vi "Stop Acquisition.vi"(0 "fpga interface in":refnum<k20>, 9 "timeout (s)":dbl=20.0 format="%#_13g", 11 "error in (no error)":errorcluster) -> (4 "fpga interface out":refnum<k20>, 15 "error out":errorcluster)   [LabVIEW 2023, in "GettingStarted_Acq_148X_Host.lvlib"]
uses:
  GettingStarted_Acq_148X_Host.lvlib
  <instrlib>/FlexRIO/CSI-2/v2/FPGA/Types/Global Acquisition Engine State.ctl
  Types/148x_Acq_FPGA_Reference.ctl
  <vilib>/Utility/error.llb/Error Cluster From Error Code.vi
  <vilib>/rvi/errors/niLvFpgaAdjustHostInterfaceError.vi
  <vilib>/rvi/interface/nirviReadWriteControl/nirviReadWriteControl.xnode
  <instrlib>/FlexRIO/CSI-2/v2/FPGA/NI CSI-2 API FPGA v2.lvlib
  NiFpgaLv.dll
  <vilib>/rvi/interface/Simulation/niFpgaSimulationCallBeginRW.vi
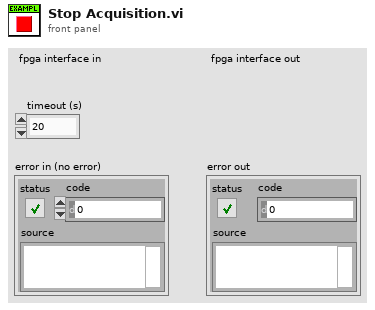
[diagram p1: front panel]
types:
  T1 = typedef "NI CSI-2 API FPGA v2.lvlib/Global Acquisition Engine State.ctl" = enum8{"Idle", "Ready For Start Trigger", "Acquire", "Error"}
  T2 = typedef "GettingStarted_Acq_148X_Host.lvlib/148x_Acq_FPGA_Reference.ctl" = refnum<k20>
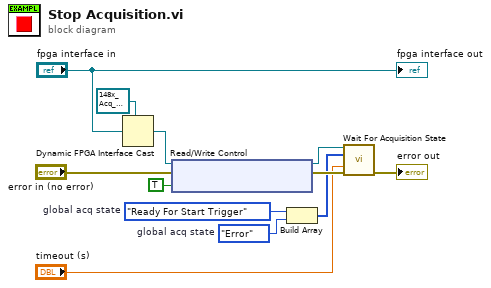
[diagram p0: block diagram]
diagram:
  w1 = Global_Acquisition_Engine_State."Error"  # global acq state
  w12 = Global_Acquisition_Engine_State."Ready For Start Trigger"  # global acq state
  n1 = Dynamic FPGA Interface Cast(Session In=T2 refnum ("FPGA VI Reference Out"), Type="fpga interface in") -> (Session Out=w4:T2)
  n2 = xnode "Read/Write Control"("FPGA VI Reference In"=w4, "error in"="error in (no error)", "sw stop trigger (strobe)"=TRUE ("stop trigger")) -> ("FPGA VI Reference Out"=w9:T2, "error out"=w10:errorcluster)
  n3 = Build Array(w12, w1) -> (w2:T1[])
  n4 = call "Wait For Acquisition State.vi"("fpga interface in"=w9, "global acq state"=w2, "timeout (s)"="timeout (s)", "error in (no error)"=w10) -> ("error out"=→"error out":errorcluster)  [unwired: 10 in, 1 out]
  "fpga interface out" <- "fpga interface in"
